vi "JPL Arm Control EX.vi"(4 "Actual Angle":dbl, 5 "Arm Control":T1, 6 "PID Settings":T3, 7 "PID Limits":cluster{"Upper Limit":dbl, "Lower Limit":dbl}) -> (0 "Arm Status":T2, 3 "output":dbl)   [LabVIEW 2015]
panel:
  out "Arm Angle Chart":dbl(graph)
  out "PID Output Chart":dbl(graph)
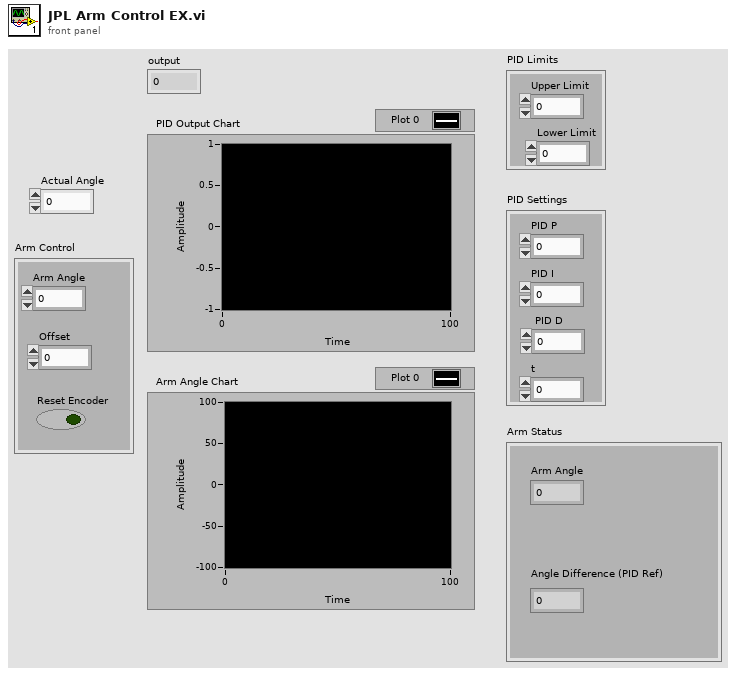
[diagram p1: front panel]
types:
  T1 = cluster{"Arm Angle":dbl, "Offset":dbl, "Reset Encoder":bool}
  T2 = cluster{"Arm Angle":dbl, "Angle Difference (PID Ref)":dbl}
  T3 = cluster{"PID P":dbl, "PID I":dbl, " PID D":dbl, "t":dbl}
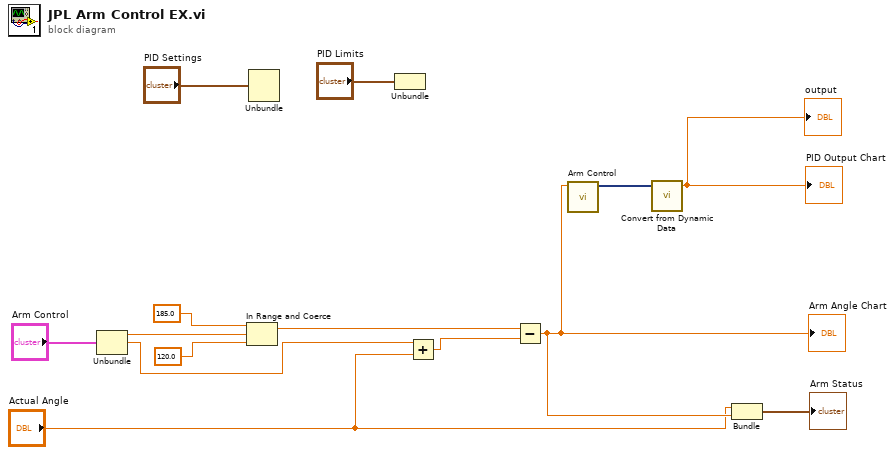
[diagram p0: block diagram]
diagram:
  n1 = Unbundle("Arm Control") -> ("Arm Angle"=w11:dbl, "Offset"=w2:dbl)  [unwired: 1 out]
  n2 = In Range and Coerce(upper limit=185.0, x=w11, lower limit=120.0) -> (coerced(x)=w8:dbl)  [unwired: 1 out]
  n3 = Unbundle("PID Settings") -> ()  [unwired: 4 out]
  n4 = Unbundle("PID Limits") -> ()  [unwired: 2 out]
  n5 = Add(x=w2, y="Actual Angle") -> (x+y=w1:dbl)
  n6 = Subtract(x=w8, y=w1) -> (x-y=w6:dbl)
  "Arm Angle Chart" <- w6
  n7 = call "Arm Control"("Signals"=w6) -> ("Scaled Signals"=w5:dynamicdata)  [unwired: 9 in, 1 out]
  n8 = call "Convert from Dynamic Data"("Dynamic Data Type"=w5) -> ("Scalar"=→"PID Output Chart" →"output":dbl)  [unwired: 3 in]
  n9 = Bundle("Actual Angle"="Actual Angle", w6) -> (→"Arm Status":cluster{"Actual Angle":dbl, dbl})  [unwired: 1 in]
